vi "Write Lifetime.vi"(8 "error in (no error)":errorcluster, 10 "Lifetime":i64, 11 "third in":refnum<class "third.lvclass">) -> (0 "error out":errorcluster, 3 "third out":refnum<class "third.lvclass">)   [LabVIEW 2015, in "third.lvclass"]
uses:
  third.lvclass
  third.lvclass/third.ctl
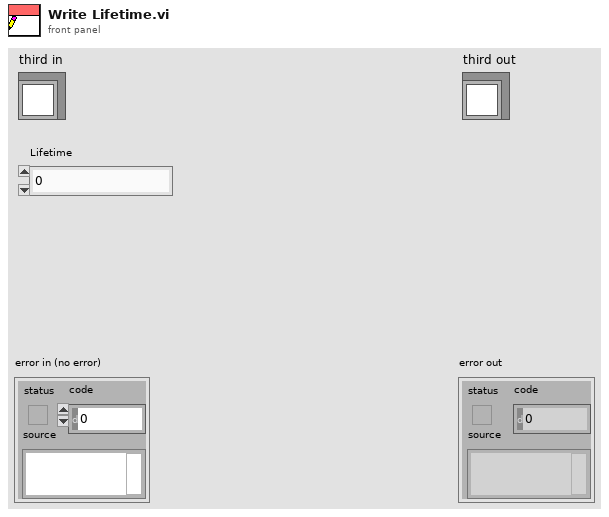
[diagram p1: front panel]
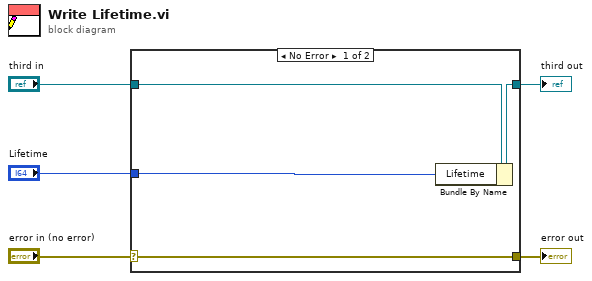
[diagram p0: block diagram]
diagram:
  n1 = case shown="No Error" "error in (no error)" {
    selector: "error in (no error)" -> [w9 w10]
    tunnel: [w9 w10] -> w4
    tunnel: [w7 w11] -> w2
    tunnel: "third in" -> [w8 w11]
    tunnel: "Lifetime" -> [w6 _]
    frame No Error {
      n2 = Bundle By Name(cluster=w8, "Lifetime"=w6) -> (w7:refnum<class "third.lvclass">)
    }
    frame Error {
    }
  }
  "error out" <- w4
  "third out" <- w2
